vi "createTitles.vi"(9 "Numeric":i32, 10 "Y axis Signal":string, 11 "X axis Signal":string) -> (3 "String":string)   [LabVIEW 2014]
doc: "André Romero - 2017\nandretec@ifsc.usp.br"
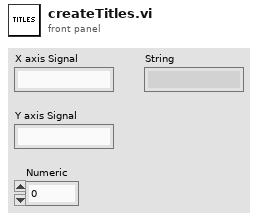
[diagram p1: front panel]
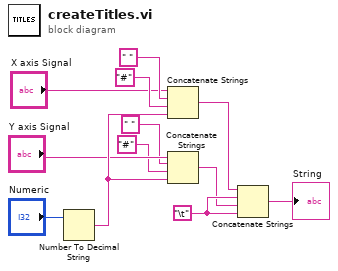
[diagram p0: block diagram]
diagram:
  w11 = "\t"
  n1 = Number To Decimal String(number="Numeric") -> (decimal integer string=w9:string)  [unwired: 1 in]
  n2 = Concatenate Strings("X axis Signal", " " ("string"), "#" ("string"), w9) -> (w5:string)
  n3 = Concatenate Strings("Y axis Signal", " " ("string"), "#" ("string"), w9) -> (w10:string)
  n4 = Concatenate Strings(w5, w11, w10, w11) -> (→"String":string)
